vi "Save Data Blocks to Binary.vi"(8 "error in":errorcluster, 9 "Block Counter In":i32, 10 "Filename":string, 11 "base path":path=path "c:/Data") -> (0 "error out":errorcluster, 1 "Block Counter Out":i32)   [LabVIEW 2012]
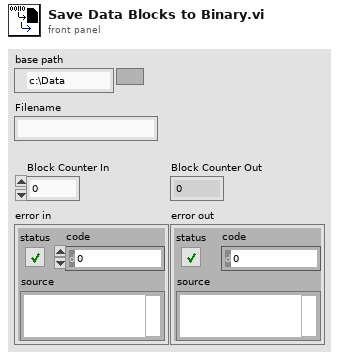
[diagram p1: front panel]
types:
  T1 = enum16{"open", "replace", "create", "open or create", "replace or create", "replace or create with confirmation"}
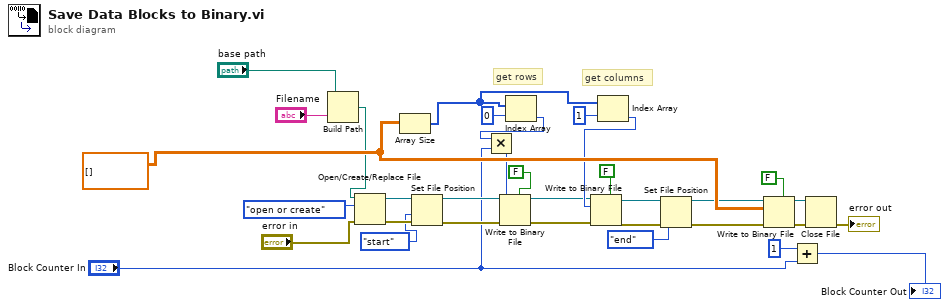
[diagram p0: block diagram]
diagram:
  w31 = dbl[][] []
  # "get columns"
  # "get rows"
  n1 = Build Path(base path="base path", name or relative path="Filename") -> (appended path=w29:path)
  n2 = Open/Create/Replace File(file path (use dialog)=w29, error in="error in", operation (0:open)=T1."open or create") -> (refnum out=w25:refnum<file>, error out=w24:errorcluster)  [unwired: 3 in, 1 out]
  n3 = Array Size(array=w31) -> (size(s)=w19:i32[])
  n4 = Set File Position(refnum=w25, from (0:start)=enum16{"start", "end", "current"}."start", error in=w24) -> (refnum out=w15:refnum<file>, error out=w16:errorcluster)  [unwired: 1 in]
  n5 = Index Array(array=w19, index=0) -> (element=w14:i32)
  n6 = Multiply(x=w14, y="Block Counter In") -> (x*y=w8:i32)
  n7 = Write to Binary File(file (use dialog)=w15, data=w8, error in=w16, 5:FALSE ("prepend array or string size? (T)")) -> (refnum out=w10:refnum<file>, error out=w12:errorcluster)  [unwired: 2 in, 1 out]
  n8 = Index Array(array=w19, index=1) -> (element=w13:i32)
  n9 = Write to Binary File(file (use dialog)=w10, data=w13, error in=w12, 5:FALSE ("prepend array or string size? (T)")) -> (refnum out=w11:refnum<file>, error out=w9:errorcluster)  [unwired: 2 in, 1 out]
  n10 = Set File Position(refnum=w11, from (0:start)=enum16{"start", "end", "current"}."end") -> (refnum out=w7:refnum<file>)  [unwired: 2 in, 1 out]
  n11 = Write to Binary File(file (use dialog)=w7, data=w31, error in=w9, 5:FALSE ("prepend array or string size? (T)")) -> (refnum out=w26:refnum<file>, error out=w27:errorcluster)  [unwired: 2 in, 1 out]
  n12 = Add(x=1, y="Block Counter In") -> (x+y=→"Block Counter Out":i32)
  n13 = Close File(refnum=w26, error in=w27) -> (error out=→"error out":errorcluster)  [unwired: 1 out]
